vi "DAQ.vi"   [LabVIEW 2017]
uses:
  C:/Users/h16034903/Downloads/Masure_Henry_projet.llb/Variable globale 1.vi
types:
  T1 = cluster{"fréquence de coupure haute passe bande":dbl, "fréquence de coupure basse passe bande":dbl, "fréquence  de coupure haute stopbande":dbl, "fréquence de coupure basse stopbande":dbl, "ordre":i32, "passebande ON":bool, "stopbande ON 2":bool}
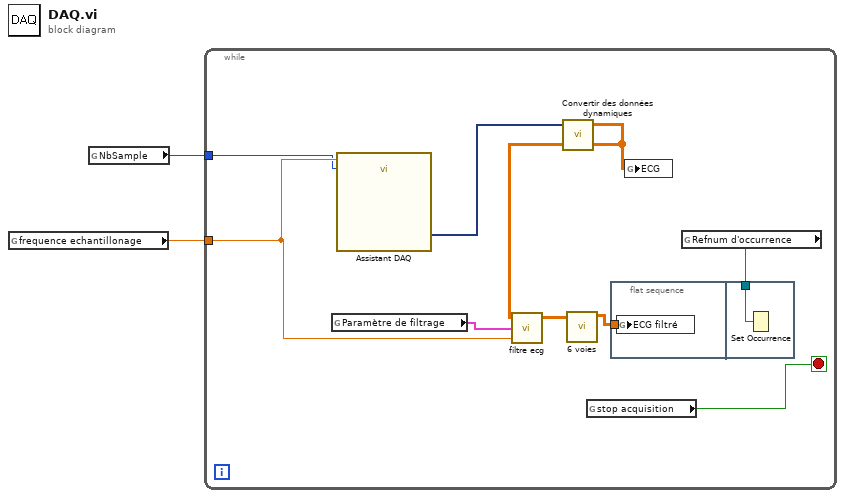
[diagram p0: block diagram]
diagram:
  n1 = global read "Variable globale 1.vi" "frequence echantillonage"() -> (w2:dbl)
  n2 = global read "Variable globale 1.vi" "NbSample"() -> (w1:i32)
  n3 = while {
    tunnel: w2 -> [w9]
    tunnel: w1 -> [w3]
    stop <- w8 stop-if-true
    n4 = global read "Variable globale 1.vi" "Paramètre de filtrage"() -> (w10:T1)
    n5 = call "Assistant DAQ"("vitesse"=w9, "nombre d'échantillons"=w3) -> ("data"=w11:dynamicdata)  [unwired: 14 in, 3 out]
    n6 = call "Convertir des données dynamiques"("Dynamic Data Type"=w11) -> ("Array"=w4:dbl[][])  [unwired: 3 in]
    n7 = call "filtre ecg.vi"("frequence echantillonage"=w9, "Paramètre de filtrage"=w10, "ECG"=w4) -> ("ECG filtré"=w7:dbl[][])  [unwired: 2 in]
    n8 = call "6 voies.vi"("ECG 2 voies"=w7) -> ("ECG à 6 voies"=w6:dbl[][])  [unwired: 10 in]
    n9 = global read "Variable globale 1.vi" "stop acquisition"() -> (w8:bool)
    n10 = flat-sequence {
      tunnel: w6 -> [w12]
      tunnel: w5 -> [w13]
      frame #0 {
        n11 = global write "Variable globale 1.vi" "ECG filtré"(w12) -> ()
      }
      frame #1 {
        n12 = Set Occurrence(w13) -> ()
      }
    }
    n13 = global write "Variable globale 1.vi" "ECG"(w4) -> ()
    n14 = global read "Variable globale 1.vi" "Refnum d'occurrence"() -> (w5:refnum<k4>)
  }
